vi "GUI_HTU_MultiCamBeamPointing1.vi"() -> ()   [LabVIEW 2020]
uses:
  Shared/GUI_Template/GUI_master/tcp_new_data_event.ctl
  Shared/GUI_Template/GUI_master/tcp new data cluster.ctl
  General GUIs/Device GUIs/GUI_Cameras/Controls/Crosshair type def.ctl
  <userlib>/_OpenG.lib/array/array.llb/Filter 1D Array with Scalar (String)__ogtk.vi
panel:
  out "x-y 8":dbl
  out "x-y 7":dbl
  out "x-y 6":dbl
  out "x-y 5":dbl
  out "x-y 4":dbl
  out "x-y 3":dbl
  out "x-y 2":dbl
  out "x-y":dbl
  out "String 8":string="x1\ny1\nx2\ny2"
  out "String 7":string="x1\ny1\nx2\ny2"
  out "String 6":string="x1\ny1\nx2\ny2"
  out "String 5":string="x1\ny1\nx2\ny2"
  out "String 4":string="x1\ny1\nx2\ny2"
  out "String 3":string="x1\ny1\nx2\ny2"
  out "String 2":string="x1\ny1\nx2\ny2"
  out "String":string="x1\ny1\nx2\ny2"
  in  "visibility":bool=TRUE
  out "appended array":string[](array[string]) caption="XH"
  out "appended array 6":string[](array[string]) caption="XH"
  out "appended array 8":string[](array[string]) caption="XH"
  out "appended array 4":string[](array[string]) caption="XH"
  in  "UDP error message":string
  out "tcp data event 2":T1
  out "error IO 2":errorcluster
  in  "Color Box":u32(colorbox)
  in  "TargetSize.Y::5":dbl=45.0 caption="y" min=2.0 max=3000.0 format="%#_6f"
  in  "TargetSize.X::5":dbl=47.0 caption="x" min=2.0 max=3000.0 format="%#_6f"
  in  "TargetSize.Y::4":dbl=45.0 caption="y" min=2.0 max=3000.0 format="%#_6f"
  in  "TargetSize.X::4":dbl=47.0 caption="x" min=2.0 max=3000.0 format="%#_6f"
  in  "TargetSize.Y::3":dbl=163.0 caption="y" min=2.0 max=3000.0 format="%#_6f"
  in  "TargetSize.X::3":dbl=152.0 caption="x" min=2.0 max=3000.0 format="%#_6f"
  in  "TargetSize.Y::2":dbl=74.0 caption="y" min=2.0 max=3000.0 format="%#_6f"
  in  "TargetSize.X::2":dbl=75.0 caption="x" min=2.0 max=3000.0 format="%#_6f"
  in  "active cams":string
  out "CCDs":string[](array[string])
  out "Cameras":T2
  in  "Target.Y::5":dbl=45.0 caption="y" min=0.0 max=2000.0 format="%#_6f"
  in  "Target.X::5":dbl=47.0 caption="x" min=0.0 max=2000.0 format="%#_6f"
  in  "Target.Y::4":dbl=45.0 caption="y" min=0.0 max=2000.0 format="%#_6f"
  in  "Target.X::4":dbl=47.0 caption="x" min=0.0 max=2000.0 format="%#_6f"
  in  "Target.Y::3":dbl=163.0 caption="y" min=0.0 max=2000.0 format="%#_6f"
  in  "Target.X::3":dbl=152.0 caption="x" min=0.0 max=2000.0 format="%#_6f"
  in  "Target.Y::2":dbl=74.0 caption="y" min=0.0 max=2000.0 format="%#_6f"
  in  "Target.X::2":dbl=75.0 caption="x" min=0.0 max=2000.0 format="%#_6f"
  out "error out":errorcluster
  in  "triggerdelay::5":dbl=0.001 caption="triggerdelay" min=10.0 max=1000000.0 format="%_4p"
  in  "triggerdelay::4":dbl=0.001 caption="triggerdelay" min=10.0 max=500000.0 format="%_4p"
  in  "triggerdelay::3":dbl=0.001 caption="triggerdelay" min=10.0 max=100000.0 format="%_4p"
  in  "triggerdelay::2":dbl=0.001 caption="triggerdelay" min=0.01 max=999000.0 format="%_4p"
  in  "trigger::5":bool caption="Trigger"
  in  "centroidy::5":dbl=0.001 caption="centroid y" min=0.0 max=0.0 format="%_4f"
  in  "centroidx::5":dbl=0.001 caption="centroid x" min=0.0 max=0.0 format="%_4f"
  in  "exposure::5":dbl=0.001 caption="exposure" min=1e-05 max=1.0 format="%_4p"
  out "image::5":T3(plugin-control) caption="HTT-MagCam-01"
  in  "GUIdevice 5":string="UC_BCaveIn"
  in  "trigger::4":bool caption="Trigger"
  in  "centroidy::4":dbl=0.001 caption="centroid y" min=0.0 max=0.0 format="%_4f"
  in  "centroidx::4":dbl=0.001 caption="centroid x" min=0.0 max=0.0 format="%_4f"
  in  "exposure::4":dbl=0.001 caption="exposure" min=5e-05 max=1.0 format="%_4p"
  out "image::4":T3(plugin-control) caption="HTT-MagCam-02"
  in  "GUIdevice 4":string="UC_DMSurface"
  in  "trigger::3":bool caption="Trigger"
  in  "centroidy::3":dbl=0.001 caption="centroid y" min=0.0 max=0.0 format="%_4f"
  in  "centroidx::3":dbl=0.001 caption="centroid x" min=0.0 max=0.0 format="%_4f"
  in  "exposure::3":dbl=0.001 caption="exposure" min=1e-05 max=1.0 format="%_4p"
  out "image::3":T3(plugin-control) caption="HTT-MagCam-03"
  in  "GUIdevice 3":string="UC_GratingMode"
  in  "trigger::2":bool caption="Trigger"
  in  "centroidy::2":dbl=0.001 min=0.0 max=0.0 format="%_4f"
  in  "centroidx::2":dbl=0.001 min=0.0 max=0.0 format="%_4f"
  in  "exposure::2":dbl=0.001 caption="exposure" min=5e-05 max=1.0 format="%_4p"
  out "image::2":T3(plugin-control) caption="HTT-MagCam-04"
  in  "GUIdevice 2":string="UC_TubeIn"
  out "tcp data event":T1
  in  "Refresh Button":bool caption="Update Crosshairs"
  in  "Select device":string(combo)="FrogHPD"
  in  "stop":bool
  in  "GUIdevice 1":string="HPD_CCD"
  # "XHair location"
  # "XHair location"
  # "XHair size"
  # "XHair size"
  # "XHair location"
  # "XHair size"
  # "XHair size"
  # "XHair location"
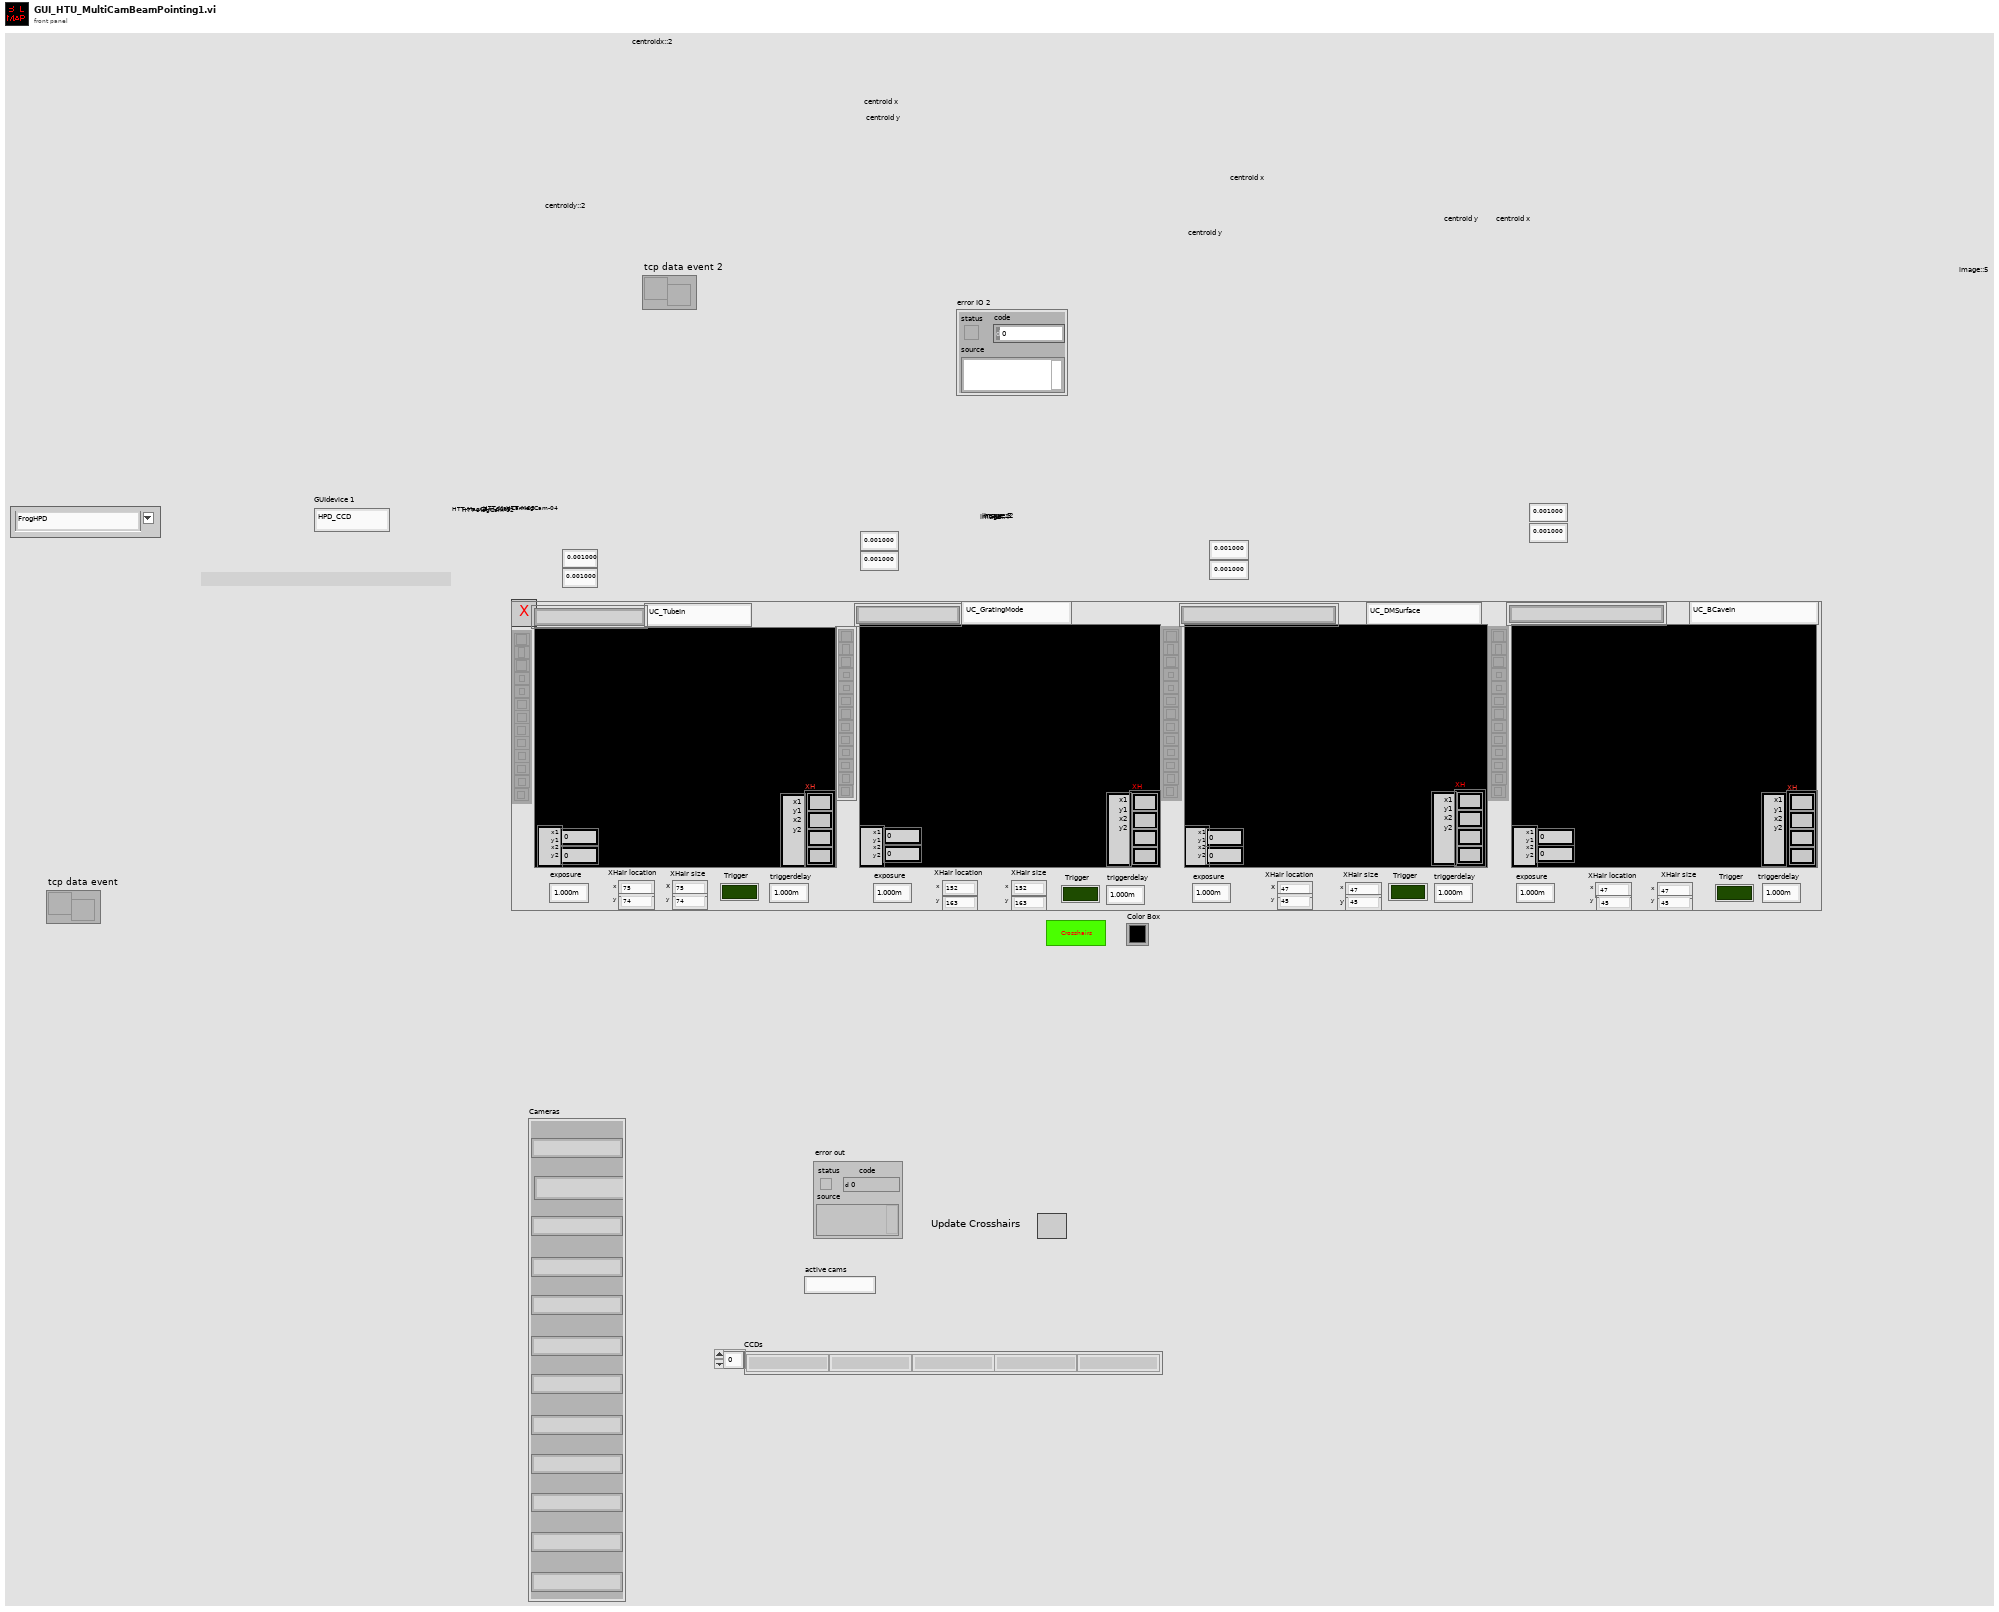
[diagram p1: front panel]
types:
  T1 = typedef "tcp_new_data_event.ctl" = refnum<user-event>
  T2 = cluster{"[0]":string, "[1]":string, "[2]":string, "[3]":string, "[4]":string, "[5]":string, "[6]":string, "[7]":string, "[8]":string, "[8] 2":string, "[8] 3":string, "[8] 4":string}
  T3 = typedef "IMAQ Image.ctl" = refnum<image>
  T4 = typedef "Image Type" = u32
  T5 = cluster{"Target.X::2":refnum<vi>, "Target.Y::2":refnum<vi>}
  T6 = cluster{"Target.X::3":refnum<vi>, "Target.Y::3":refnum<vi>}
  T7 = cluster{"Target.X::4":refnum<vi>, "Target.Y::4":refnum<vi>}
  T8 = cluster{"Target.X::5":refnum<vi>, "Target.Y::5":refnum<vi>}
  T9 = cluster{"TargetSize.X::2":refnum<vi>, "TargetSize.Y::2":refnum<vi>}
  T10 = cluster{"TargetSize.X::3":refnum<vi>, "TargetSize.Y::3":refnum<vi>}
  T11 = cluster{"TargetSize.X::4":refnum<vi>, "TargetSize.Y::4":refnum<vi>}
  T12 = cluster{"TargetSize.X::5":refnum<vi>, "TargetSize.Y::5":refnum<vi>}
  T13 = cluster{"Target.X::5":refnum<vi>, "Target.Y::5":refnum<vi>}[]
  T14 = cluster{"TargetSize.X::5":refnum<vi>, "TargetSize.Y::5":refnum<vi>}[]
  T15 = cluster{"[0]":string, "[1]":string, "[2]":string, "[3]":string, "[4]":string, "[5]":string, "[6]":string, "[7]":string, "[8]":string, "[9]":string, "[10]":string, "[11]":string}
  T16 = typedef "Crosshair type def.ctl" = cluster{"Draw":bool, "Target":cluster{"x":dbl, "y":dbl}, "Size":cluster{"x":dbl, "y":dbl}, "Angle":dbl, "Color":u32, "Thickness":u8, "CrosshairLabel":string}
  T17 = cluster{"Left":i32, "Top":i32, "Right":i32, "Bottom":i32}
  T18 = enum32{"invalid app kind", "Development System", "Run Time System", "Student Edition", "Embedded LabVIEW", "Evaluation", "Custom"}
  T19 = typedef "tcp new data cluster.ctl" = cluster{"EventEnum":enum16{"new data", "connection status update"}, "Device name":string}
  T20 = enum32{"Invalid", "Standard", "Closed", "Hidden", "Minimized", "Maximized"}
  T21 = cluster{"Core":cluster{"Current VI Reference":refnum<vi>, "Close Panel on Exit?":bool}, "Your Boolean data":bool, "active cams":string, "SuperGUI":cluster{"STOP queue":refnum<queue>, "SuperGUI ref":refnum<vi>}}
  T22 = cluster{"STOP queue":refnum<queue>, "SuperGUI ref":refnum<vi>}
  T23 = cluster{"Current VI Reference":refnum<vi>, "Close Panel on Exit?":bool}
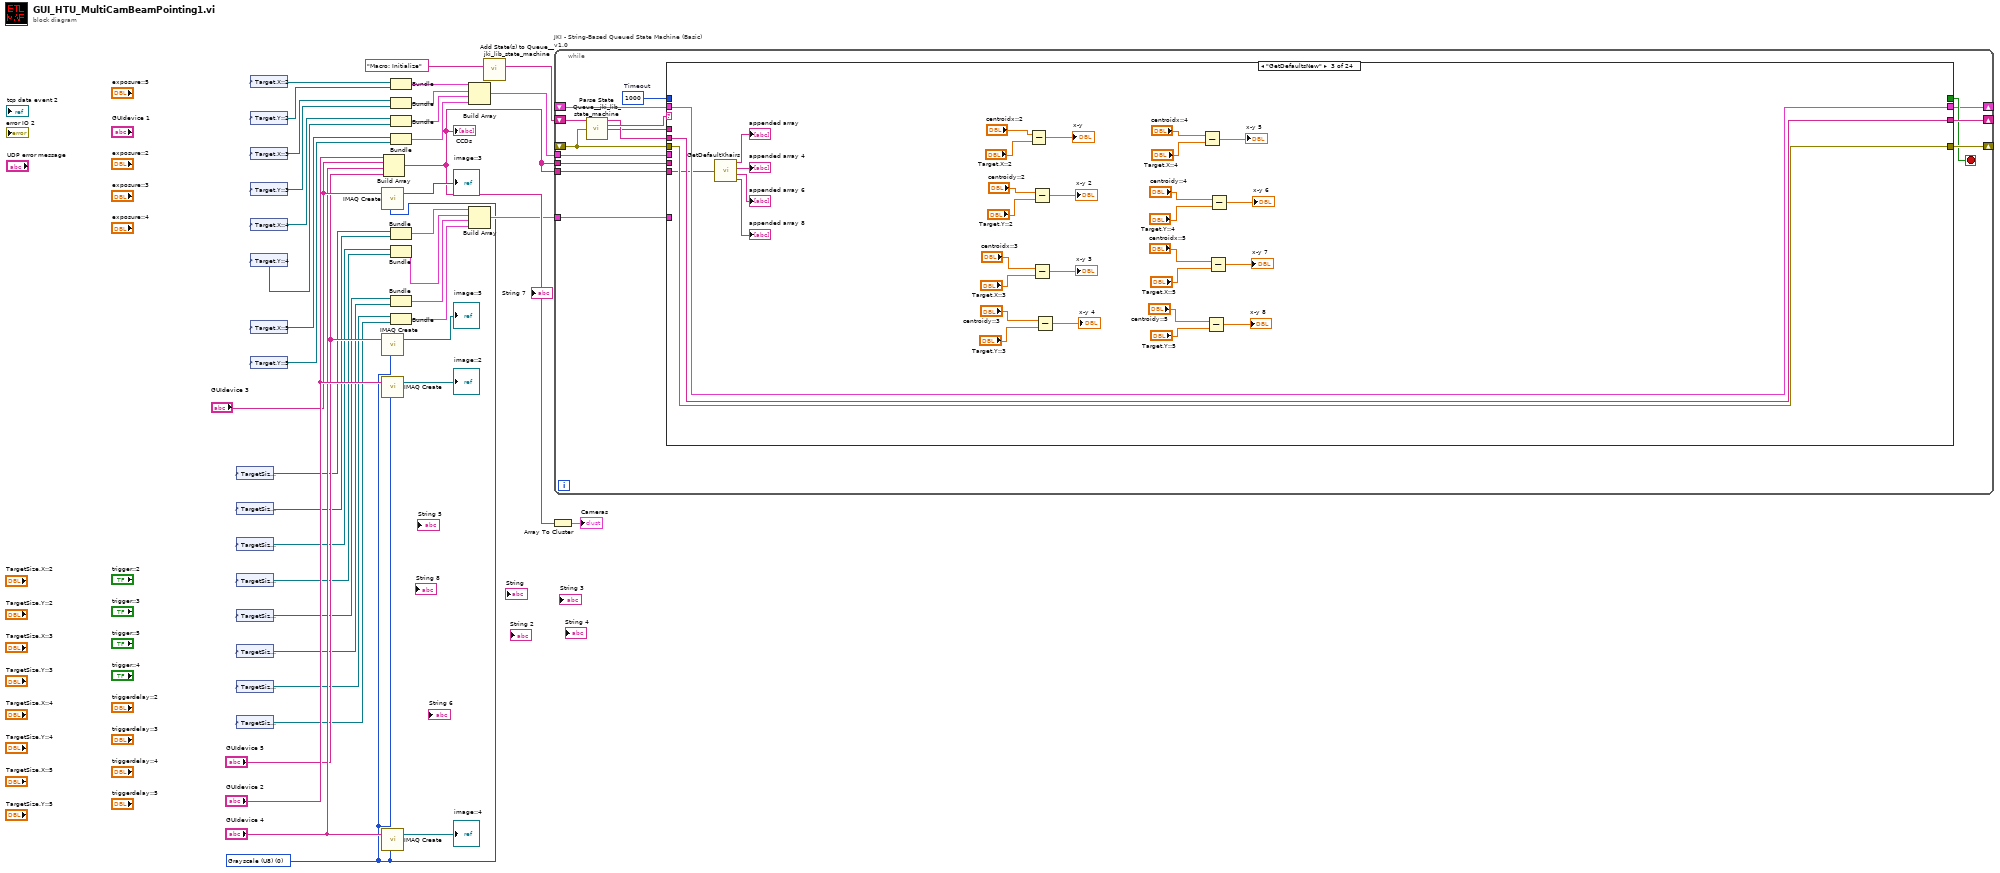
[diagram p0: block diagram]
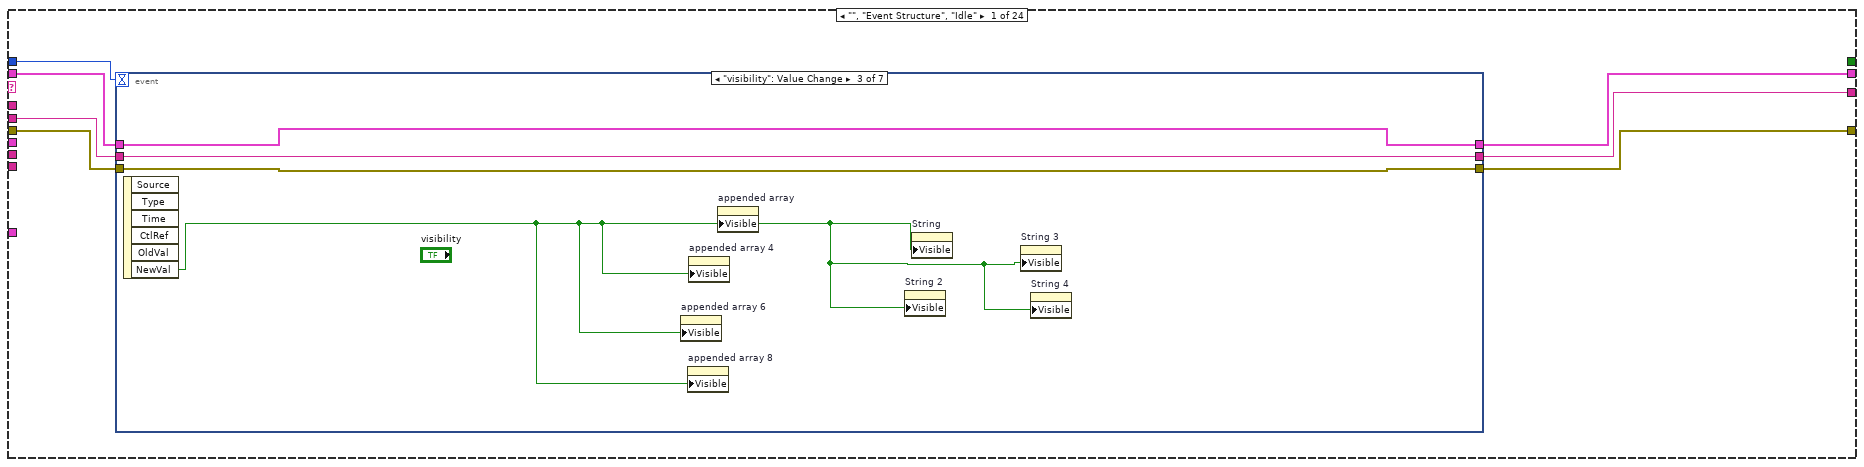
[diagram p2: hidden frame]
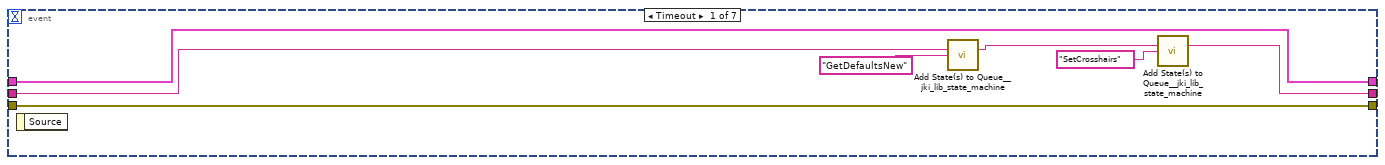
[diagram p3: hidden frame]
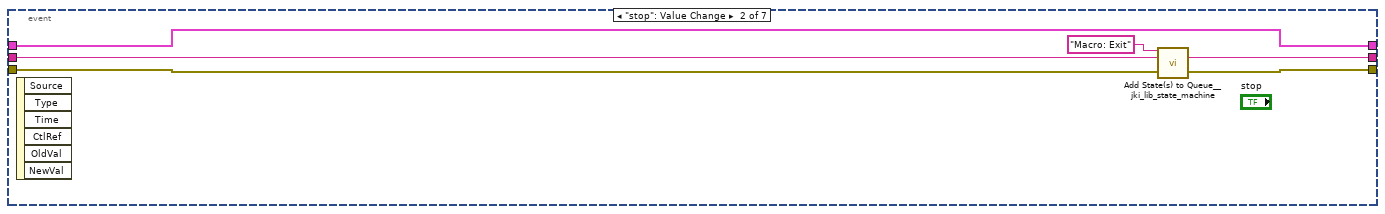
[diagram p4: hidden frame]
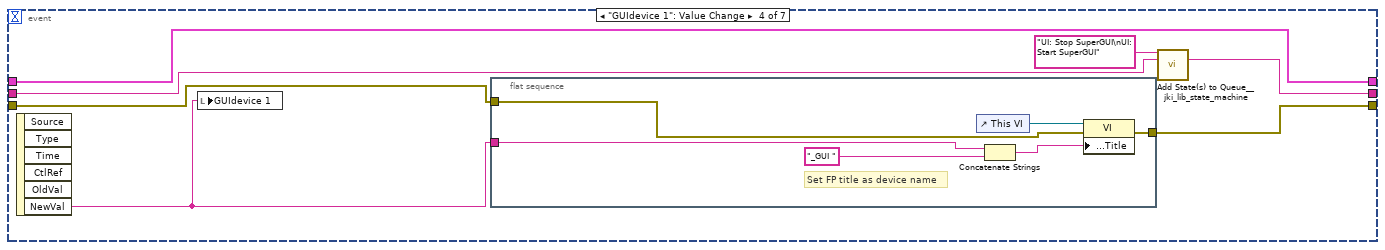
[diagram p5: hidden frame]
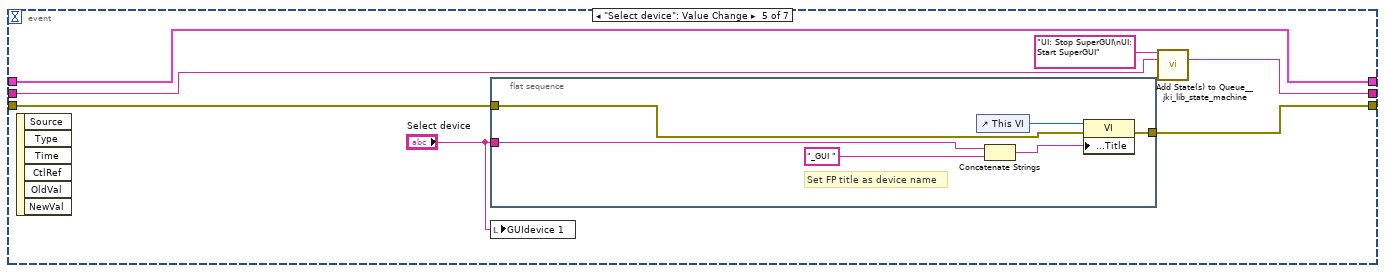
[diagram p6: hidden frame]
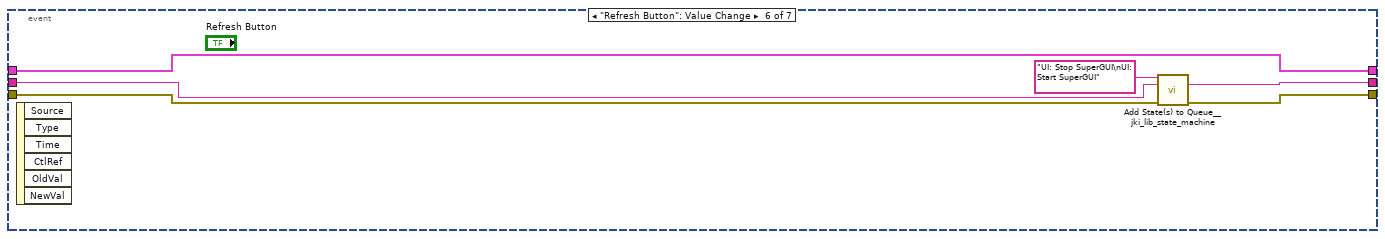
[diagram p7: hidden frame]
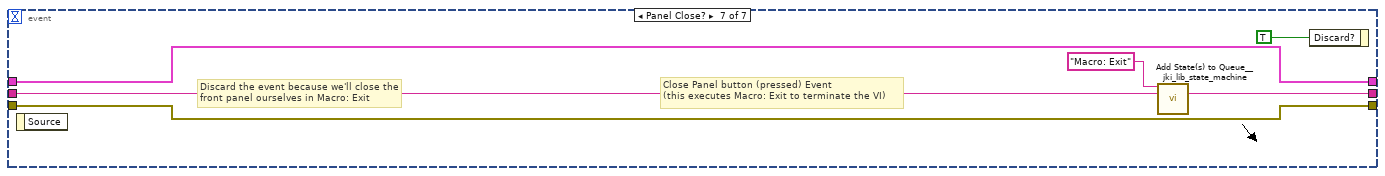
[diagram p8: hidden frame]
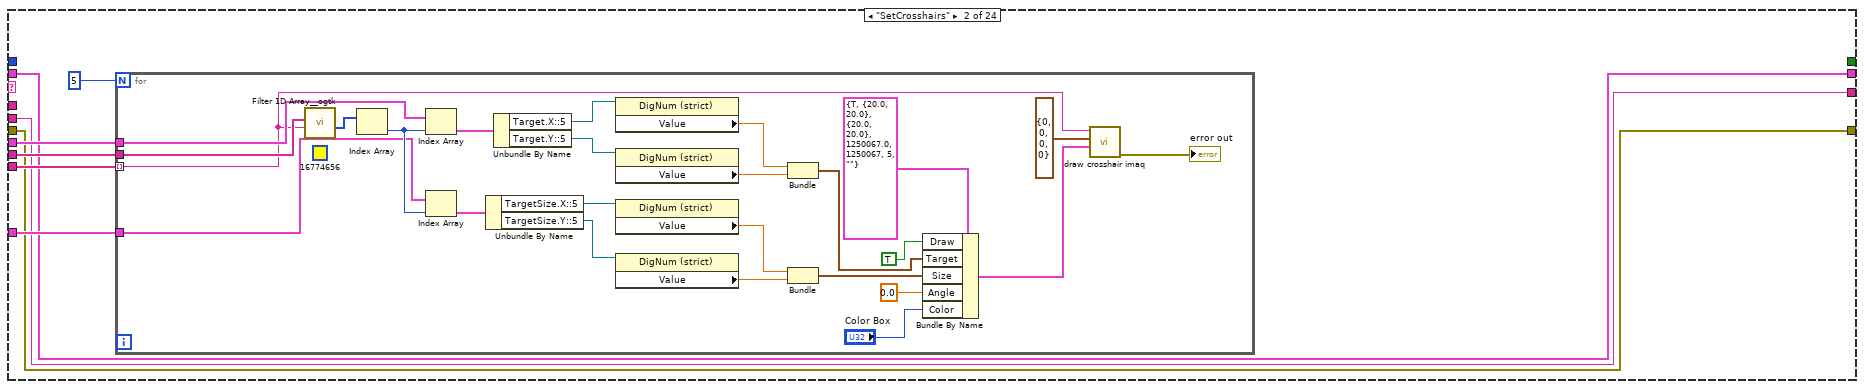
[diagram p9: hidden frame]
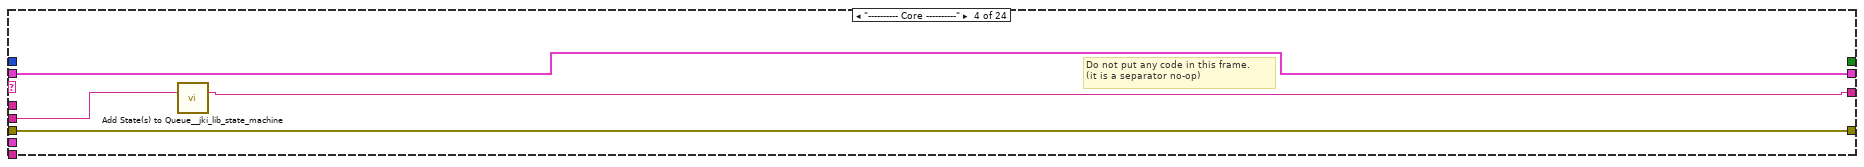
[diagram p10: hidden frame]
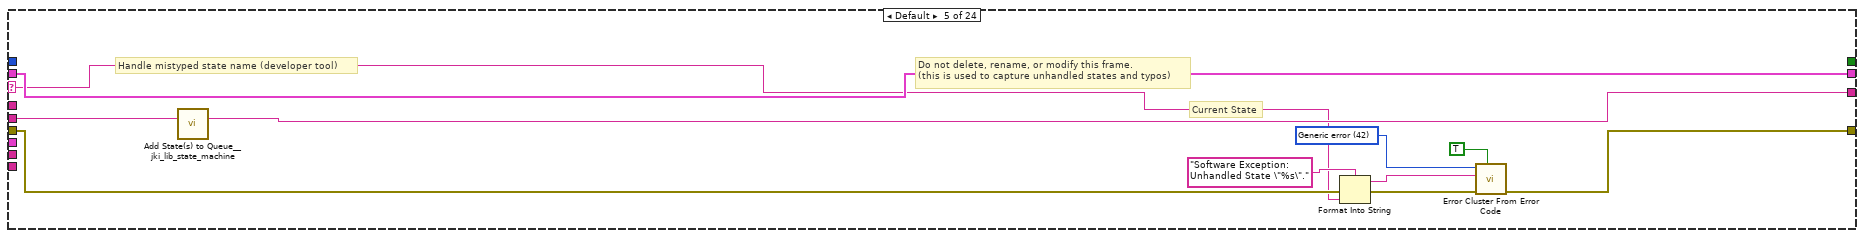
[diagram p11: hidden frame]
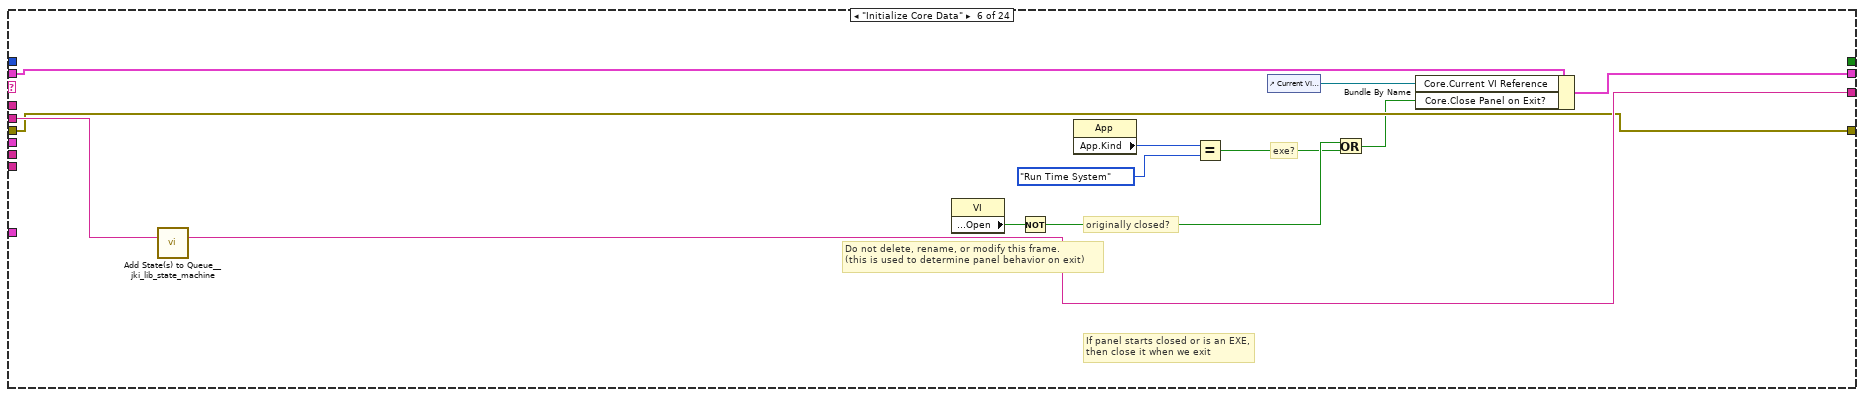
[diagram p12: hidden frame]
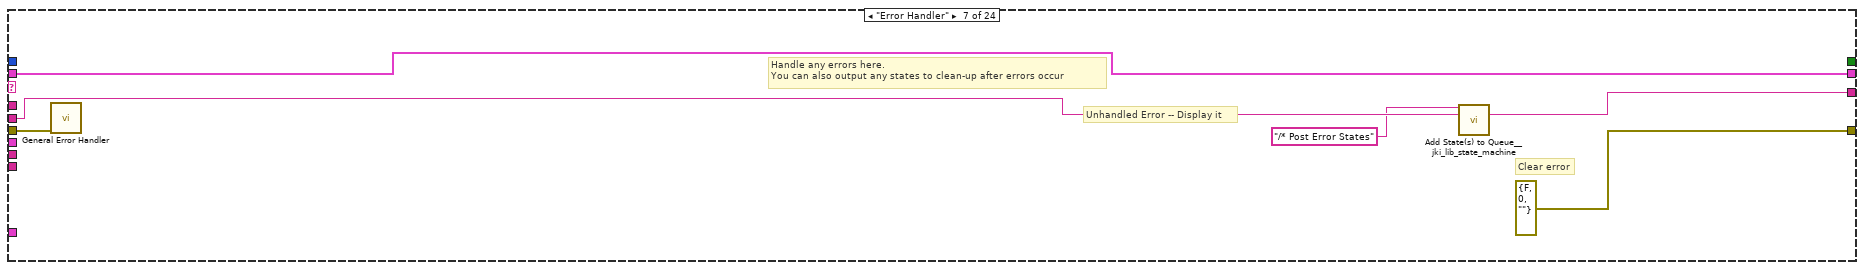
[diagram p13: hidden frame]
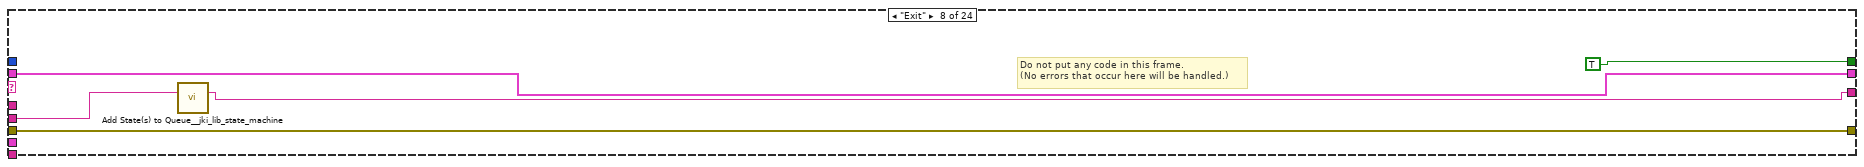
[diagram p14: hidden frame]
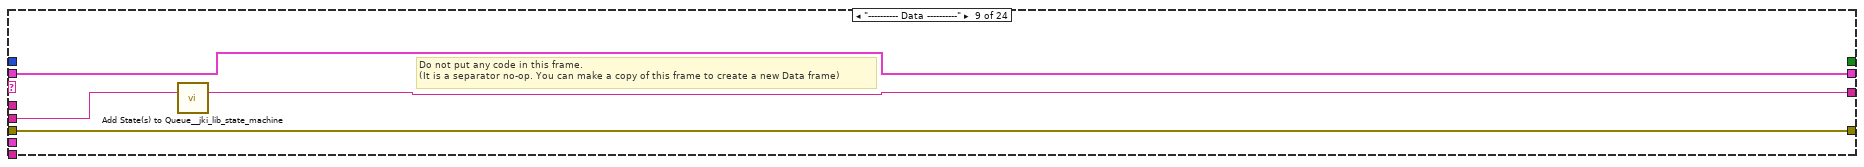
[diagram p15: hidden frame]
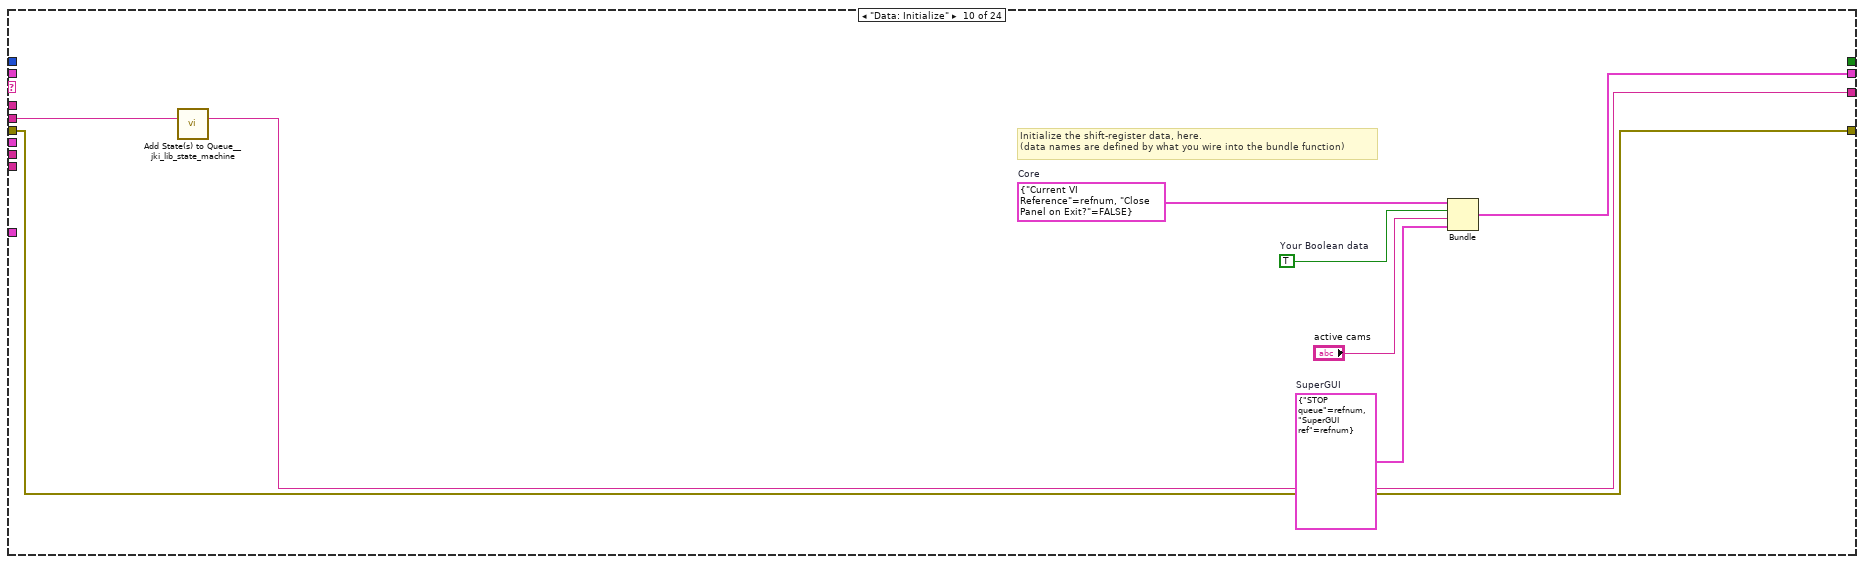
[diagram p16: hidden frame]
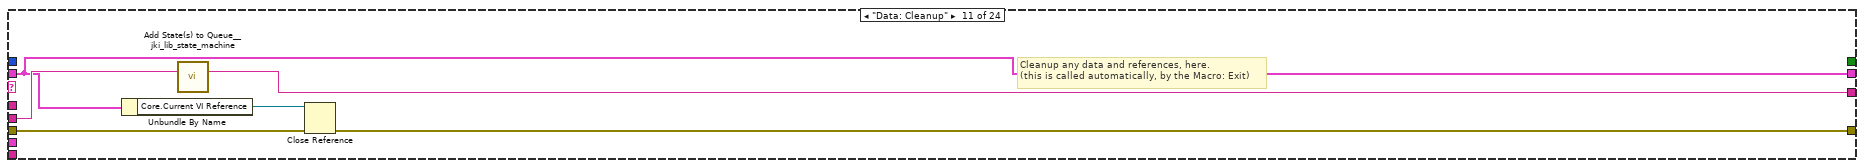
[diagram p17: hidden frame]
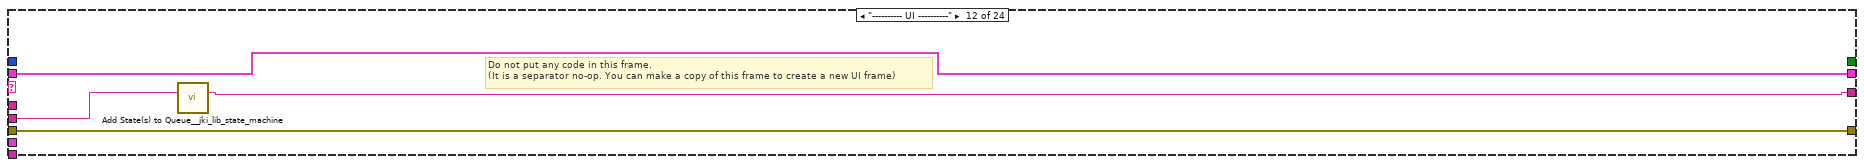
[diagram p18: hidden frame]
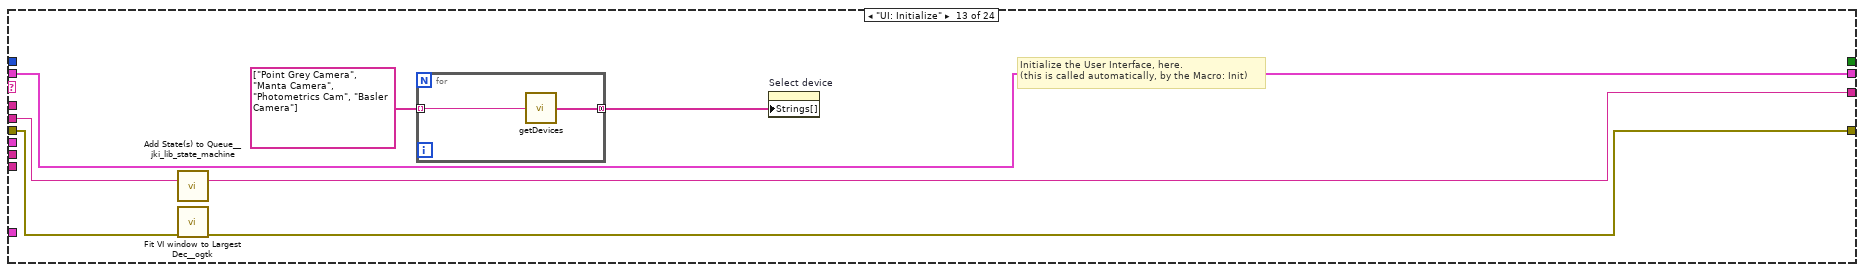
[diagram p19: hidden frame]
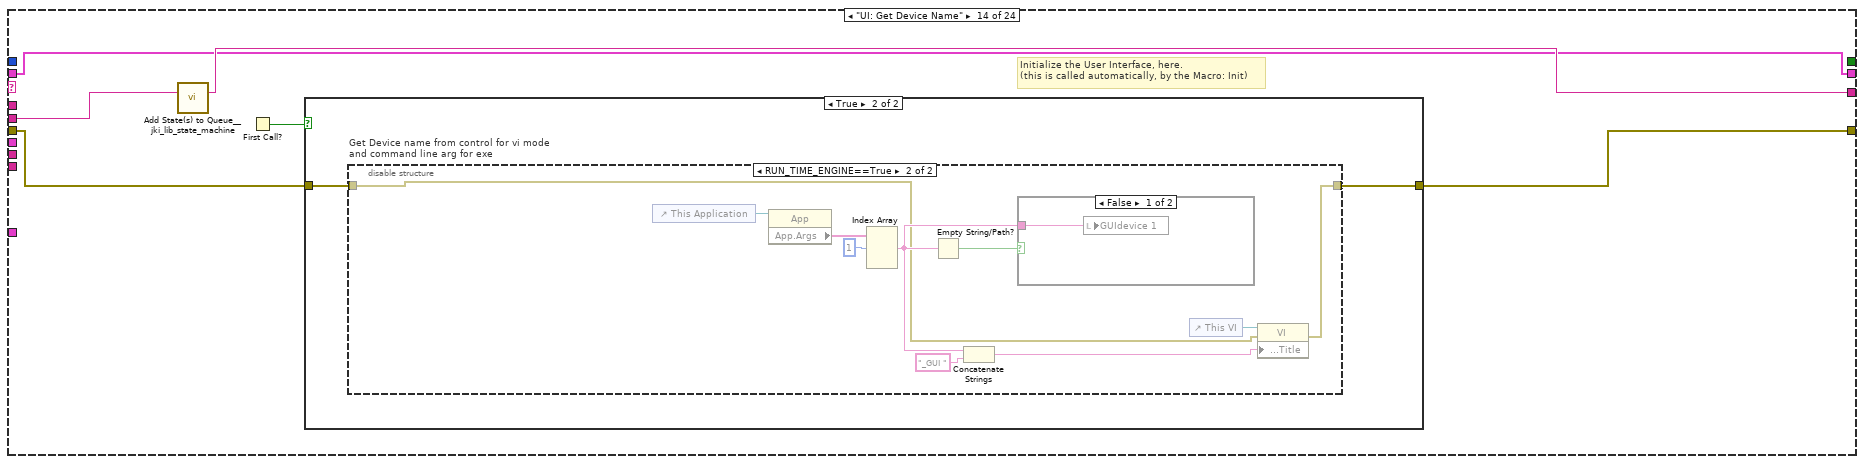
[diagram p20: hidden frame]
diagram:
  w1 = T4 0 items=["Grayscale (U8)", "Grayscale (I16)", "Grayscale (SGL)", "Complex (CSG)", "RGB (U32)", "HSL (U32)", "RGB (U64)", "Grayscale (U16)"] ("Image Type")
  n1 = control-ref of="TargetSize.X::2"() -> (w14:refnum<vi>)
  n2 = control-ref of="TargetSize.Y::2"() -> (w13:refnum<vi>)
  n3 = control-ref of="TargetSize.X::3"() -> (w12:refnum<vi>)
  n4 = control-ref of="TargetSize.Y::3"() -> (w11:refnum<vi>)
  n5 = control-ref of="TargetSize.X::4"() -> (w10:refnum<vi>)
  n6 = control-ref of="TargetSize.Y::4"() -> (w9:refnum<vi>)
  n7 = control-ref of="TargetSize.X::5"() -> (w8:refnum<vi>)
  n8 = control-ref of="TargetSize.Y::5"() -> (w7:refnum<vi>)
  n9 = control-ref of="Target.X::2"() -> (w33:refnum<vi>)
  n10 = control-ref of="Target.Y::2"() -> (w32:refnum<vi>)
  n11 = control-ref of="Target.X::3"() -> (w31:refnum<vi>)
  n12 = control-ref of="Target.Y::3"() -> (w30:refnum<vi>)
  n13 = control-ref of="Target.X::4"() -> (w29:refnum<vi>)
  n14 = control-ref of="Target.Y::4"() -> (w28:refnum<vi>)
  n15 = control-ref of="Target.X::5"() -> (w27:refnum<vi>)
  n16 = control-ref of="Target.Y::5"() -> (w26:refnum<vi>)
  n17 = call "IMAQ Create"("Image Name"="GUIdevice 3", "Image Type"=w1) -> ("New Image"=→"image::3":T3)  [unwired: 3 in, 1 out]
  n18 = call "IMAQ Create"("Image Name"="GUIdevice 5", "Image Type"=w1) -> ("New Image"=→"image::5":T3)  [unwired: 3 in, 1 out]
  n19 = call "IMAQ Create"("Image Name"="GUIdevice 2", "Image Type"=w1) -> ("New Image"=→"image::2":T3)  [unwired: 3 in, 1 out]
  n20 = call "IMAQ Create"("Image Name"="GUIdevice 4", "Image Type"=w1) -> ("New Image"=→"image::4":T3)  [unwired: 3 in, 1 out]
  n21 = Build Array("GUIdevice 2", "GUIdevice 3", "GUIdevice 4", "GUIdevice 5") -> (w15:string[])
  "CCDs" <- w15
  n22 = Bundle("Target.X::2"=w33, "Target.Y::2"=w32) -> (w25:T5)  [unwired: 1 in]
  n23 = Bundle("Target.X::3"=w31, "Target.Y::3"=w30) -> (w24:T6)  [unwired: 1 in]
  n24 = Bundle("Target.X::4"=w29, "Target.Y::4"=w28) -> (w22:T7)  [unwired: 1 in]
  n25 = Bundle("Target.X::5"=w27, "Target.Y::5"=w26) -> (w23:T8)  [unwired: 1 in]
  n26 = Bundle("TargetSize.X::2"=w14, "TargetSize.Y::2"=w13) -> (w6:T9)  [unwired: 1 in]
  n27 = Bundle("TargetSize.X::3"=w12, "TargetSize.Y::3"=w11) -> (w5:T10)  [unwired: 1 in]
  n28 = Bundle("TargetSize.X::4"=w10, "TargetSize.Y::4"=w9) -> (w3:T11)  [unwired: 1 in]
  n29 = Bundle("TargetSize.X::5"=w8, "TargetSize.Y::5"=w7) -> (w4:T12)  [unwired: 1 in]
  n30 = Build Array(w25, w24, w22, w23) -> (w21:T13)
  n31 = Build Array(w6, w5, w3, w4) -> (w2:T14)
  n32 = call <vilib>:"Add State(s) to Queue__jki_lib_state_machine.vi"("State(s) in (\"\")"="Macro: Initialize") -> ("States Out"=w39:string)  [unwired: 14 in]
  n33 = Array To Cluster(array=w15) -> (cluster=→"Cameras":T15)
  n34 = while "JKI - String-Based Queued State Machine (Basic) v1.0" {
    shift-right: [w47] -> _
    shift-left: _ -> [w44]
    shift-right: [w50] -> _
    shift-left: _ -> [w45]
    shift-right: [w49] -> _
    shift-left: w39 -> [w51]
    tunnel: w21 -> [w41]
    tunnel: w15 -> [w42]
    tunnel: w15 -> [w43]
    tunnel: w2 -> [w40]
    stop <- w48 stop-if-true
    w46 = 1000  # Timeout
    n35 = call <vilib>:"Parse State Queue__jki_lib_state_machine.vi"("State Queue"=w51, "Error In (no error)"=w45) -> ("Remaining States"=w53:string, "Current State"=w54:string, "Arguments"=w52:string)  [unwired: 11 in]
    n36 = case shown="\"GetDefaultsNew\"" w54 {
      selector: w54 -> [_ _ _ _ w184 _ _ _ _ _ _ _ _ _ _ _ _ _ _ _ _ _ _ _]
      tunnel: w53 -> [w61 w117 w178 w183 w188 w206 w212 w217 w221 w229 w235 w239 w246 w254 w289 w297 w303 w314 w340 w345 w355 w359 w363 w367]
      tunnel: w52 -> [_ _ _ _ _ _ _ _ _ _ _ _ _ _ _ _ w298 w308 _ _ _ _ _ _]
      tunnel: w44 -> [w59 w118 w179 w180 w186 w197 w209 w215 w218 _ w230 w236 w244 w252 w280 w292 w301 w310 w337 w342 w352 w356 w360 w364]
      tunnel: [w58 w116 w177 w181 w190 w203 errorcluster {"status"=FALSE, "code"=0, "source"=""} ("error out") w214 w219 w226 w231 w237 w242 w249 w273 w290 w299 w311 w338 w343 w353 w357 w361 w365] -> w50
      tunnel: w45 -> [w57 w116 w177 w181 w189 w203 w208 w214 w219 w226 w232 w237 w243 w250 w274 w291 w300 w312 w338 w343 w353 w357 w361 w365]
      tunnel: [w60 w117 w178 w182 w187 w205 w211 w216 w220 w228 w234 w238 w245 w253 w288 w296 w302 w313 w339 w344 w354 w358 w362 w366] -> w49
      tunnel: [_ _ _ _ _ _ _ TRUE _ _ _ _ _ _ _ _ _ _ _ _ _ _ _ _] -> w48
      tunnel: [w56 w118 w179 w180 w186 w204 w209 w215 w218 w227 w230 w236 w244 w252 w279 w292 w301 w310 w337 w342 w352 w356 w360 w364] -> w47
      tunnel: w46 -> [w55 _ _ _ _ _ _ _ _ _ _ _ _ _ _ _ _ _ _ _ _ _ _ _]
      tunnel: w43 -> [_ w120 w176 _ _ _ _ _ _ _ _ _ _ _ _ _ _ _ _ _ _ _ _ _]
      tunnel: w42 -> [_ w121 _ _ _ _ _ _ _ _ _ _ _ _ _ _ _ _ _ _ _ _ _ _]
      tunnel: w41 -> [_ w122 _ _ _ _ _ _ _ _ _ _ _ _ _ _ _ _ _ _ _ _ _ _]
      tunnel: w40 -> [_ w119 _ _ _ _ _ _ _ _ _ _ _ _ _ _ _ _ _ _ _ _ _ _]
      frame "", "Event Structure", "Idle" {
        n37 = event shown="[2] \"visibility\": Value Change" {
          selector: _ -> [_ _ _ _ _ _ _]
          dyn-events: _ -> [_ _ _ _ _ _ _]
          timeout: w55 -> [_ _ _ _ _ _ _]
          tunnel: w61 -> [w64 w71 w75 w81 w93 w106 w114]
          tunnel: [w68 w70 w75 w80 w92 w105 w113] -> w60
          tunnel: w59 -> [w66 w73 w77 w84 w97 w108 w111]
          tunnel: [w67 w72 w76 w82 w95 w107 w112] -> w58
          tunnel: w57 -> [w67 w72 w76 w83 w96 w107 w112]
          tunnel: [w66 w73 w77 w84 w97 w108 w111] -> w56
          event Timeout {
            n38 = event-data() -> ()  [unwired: 1 in, 1 out]
            n39 = call <vilib>:"Add State(s) to Queue__jki_lib_state_machine.vi"("State(s) in (\"\")"=w64, "State(s) at Back (\"\")"="GetDefaultsNew") -> ("States Out"=w62:string)  [unwired: 13 in]
            n40 = call <vilib>:"Add State(s) to Queue__jki_lib_state_machine.vi"("State(s) in (\"\")"=w62, "State(s) at Back (\"\")"="SetCrosshairs") -> ("States Out"=w68:string)  [unwired: 13 in]
          }
          event "stop": Value Change {
            n41 = event-data() -> ()  [unwired: 1 in, 6 out]
            n42 = call <vilib>:"Add State(s) to Queue__jki_lib_state_machine.vi"("State(s) in Front (\"\")"="Macro: Exit", "State(s) in (\"\")"=w71) -> ("States Out"=w70:string)  [unwired: 13 in]
          }
          event "visibility": Value Change {
            n43 = event-data() -> ("NewVal"=w74:bool)  [unwired: 1 in, 5 out]
            n44 = property on="appended array 6" class="Arr (strict)"("Visible"=w74) -> ()  [unwired: 2 in, 2 out]
            n45 = property on="appended array 8" class="Arr (strict)"("Visible"=w74) -> ()  [unwired: 2 in, 2 out]
            n46 = property on="appended array 4" class="Arr (strict)"("Visible"=w74) -> ()  [unwired: 2 in, 2 out]
            n47 = property on="appended array" class="Arr (strict)"("Visible"=w74) -> ()  [unwired: 2 in, 2 out]
            n48 = property on="String 2" class="Str"("Visible"=w74) -> ()  [unwired: 2 in, 2 out]
            n49 = property on="String" class="Str"("Visible"=w74) -> ()  [unwired: 2 in, 2 out]
            n50 = property on="String 3" class="Str"("Visible"=w74) -> ()  [unwired: 2 in, 2 out]
            n51 = property on="String 4" class="Str"("Visible"=w74) -> ()  [unwired: 2 in, 2 out]
          }
          event "GUIdevice 1": Value Change {
            n52 = event-data() -> ("NewVal"=w78:string)  [unwired: 1 in, 5 out]
            n53 = local write "GUIdevice 1"(w78) -> ()
            n54 = flat-sequence {
              tunnel: [w87] -> w82
              tunnel: w83 -> [w86]
              tunnel: w78 -> [w85]
              frame #0 {
                # "Set FP title as device name"
                n55 = control-ref of="This VI"() -> (w90:refnum<vi>)
                n56 = Concatenate Strings(w85, "_GUI ") -> (w89:string)
                n57 = property class="VI"(reference=w90, error in=w86, "Front Panel.Title"=w89) -> (error out=w87:errorcluster)  [unwired: 1 out]
              }
            }
            n58 = call <vilib>:"Add State(s) to Queue__jki_lib_state_machine.vi"("State(s) in Front (\"\")"="UI: Stop SuperGUI\nUI: Start SuperGUI", "State(s) in (\"\")"=w81) -> ("States Out"=w80:string)  [unwired: 13 in]
          }
          event "Select device": Value Change {
            n59 = event-data() -> ()  [unwired: 1 in, 6 out]
            n60 = flat-sequence {
              tunnel: [w100] -> w95
              tunnel: w96 -> [w99]
              tunnel: "Select device" -> [w98]
              frame #0 {
                # "Set FP title as device name"
                n61 = control-ref of="This VI"() -> (w103:refnum<vi>)
                n62 = Concatenate Strings(w98, "_GUI ") -> (w102:string)
                n63 = property class="VI"(reference=w103, error in=w99, "Front Panel.Title"=w102) -> (error out=w100:errorcluster)  [unwired: 1 out]
              }
            }
            n64 = local write "GUIdevice 1"("Select device") -> ()
            n65 = call <vilib>:"Add State(s) to Queue__jki_lib_state_machine.vi"("State(s) in Front (\"\")"="UI: Stop SuperGUI\nUI: Start SuperGUI", "State(s) in (\"\")"=w93) -> ("States Out"=w92:string)  [unwired: 13 in]
          }
          event "Refresh Button": Value Change {
            n66 = event-data() -> ()  [unwired: 1 in, 6 out]
            n67 = call <vilib>:"Add State(s) to Queue__jki_lib_state_machine.vi"("State(s) in Front (\"\")"="UI: Stop SuperGUI\nUI: Start SuperGUI", "State(s) in (\"\")"=w106) -> ("States Out"=w105:string)  [unwired: 13 in]
          }
          event Panel Close? {
            # "Discard the event because we'll close the front panel ourselves in Macro: Exit"
            # "Close Panel button (pressed) Event\n(this executes Macro: Exit to terminate the VI)"
            n68 = event-data() -> ()  [unwired: 1 in, 1 out]
            n69 = call <vilib>:"Add State(s) to Queue__jki_lib_state_machine.vi"("State(s) in Front (\"\")"="Macro: Exit", "State(s) in (\"\")"=w114) -> ("States Out"=w113:string)  [unwired: 13 in]
            n70 = event-data("Discard?"=TRUE) -> ()  [unwired: 1 in, 1 out]
          }
        }
      }
      frame "SetCrosshairs" {
        n71 = for {
          N: 5 -> [_]
          tunnel: w121 -> [w126]
          tunnel: w122 -> [w125]
          tunnel: w119 -> [w124]
          tunnel: w120 -> [w123] mode=indexing
          (unwired) u32 16774656 ("Color")
          n72 = call-poly <userlib>:"Filter 1D Array__ogtk.vi"("items to filter"=w123, "array"=w126) -> ("filtered item indices"=w130:i32[])  [unwired: 4 in, 1 out]
          n73 = Index Array(array=w130) -> (element=w133:i32)  [unwired: 1 in]
          n74 = Index Array(array=w125, index=w133) -> (element=w131:T8)
          n75 = Index Array(array=w124, index=w133) -> (element=w134:T12)
          n76 = Unbundle By Name(w134) -> ("TargetSize.X::5"=w135:refnum<vi>, "TargetSize.Y::5"=w136:refnum<vi>)
          n77 = Unbundle By Name(w131) -> ("Target.X::5"=w128:refnum<vi>, "Target.Y::5"=w129:refnum<vi>)
          n78 = property class="DigNum (strict)"(reference=w128) -> ("Value"=w142:dbl)  [unwired: 1 in, 2 out]
          n79 = property class="DigNum (strict)"(reference=w129) -> ("Value"=w143:dbl)  [unwired: 1 in, 2 out]
          n80 = property class="DigNum (strict)"(reference=w135) -> ("Value"=w137:dbl)  [unwired: 1 in, 2 out]
          n81 = property class="DigNum (strict)"(reference=w136) -> ("Value"=w138:dbl)  [unwired: 1 in, 2 out]
          n82 = Bundle("Value"=w142, "Value"=w143) -> (w144:cluster{"Value":dbl, "Value":dbl})  [unwired: 1 in]
          n83 = Bundle("Value"=w137, "Value"=w138) -> (w145:cluster{"Value":dbl, "Value":dbl})  [unwired: 1 in]
          n84 = Bundle By Name(cluster=T16 {"Draw"=TRUE, "Target"={"x"=20.0, "y"=20.0}, "Size"={"x"=20.0, "y"=20.0}, "Angle"=1250067.0, "Color"=1250067, "Thickness"=5, "CrosshairLabel"=""} ("Crosshair"), "Draw"=TRUE, "Target"=w144, "Size"=w145, "Angle"=0.0, "Color"="Color Box") -> (w140:T16)
          n85 = call "draw crosshair imaq.vi"("Crosshair"=w140, "Bounding Rectangle"=T17 {"Left"=0, "Top"=0, "Right"=0, "Bottom"=0}, "image in"=w123) -> ("error out"=→"error out":errorcluster)  [unwired: 7 in, 1 out]
        }
      }
      frame "GetDefaultsNew" {
        n86 = call "GetDefaultXhairs.vi"("appended array 2"=w176) -> ("appended array"=→"appended array":string[], "appended array 4"=→"appended array 4":string[], "appended array 6"=→"appended array 6":string[], "appended array 8"=→"appended array 8":string[])
        n87 = Subtract(x="centroidx::2", y="Target.X::2") -> (x-y=→"x-y":dbl)
        n88 = Subtract(x="centroidy::2", y="Target.Y::2") -> (x-y=→"x-y 2":dbl)
        n89 = Subtract(x="centroidx::3", y="Target.X::3") -> (x-y=→"x-y 3":dbl)
        n90 = Subtract(x="centroidy::3", y="Target.Y::3") -> (x-y=→"x-y 4":dbl)
        n91 = Subtract(x="centroidx::4", y="Target.X::4") -> (x-y=→"x-y 5":dbl)
        n92 = Subtract(x="centroidy::5", y="Target.Y::5") -> (x-y=→"x-y 8":dbl)
        n93 = Subtract(x="centroidx::5", y="Target.X::5") -> (x-y=→"x-y 7":dbl)
        n94 = Subtract(x="centroidy::4", y="Target.Y::4") -> (x-y=→"x-y 6":dbl)
      }
      frame "---------- Core ----------" {
        # "Do not put any code in this frame.\n(it is a separator no-op)"
        n95 = call <vilib>:"Add State(s) to Queue__jki_lib_state_machine.vi"("State(s) in (\"\")"=w183) -> ("States Out"=w182:string)  [unwired: 14 in]
      }
      frame Default {
        w193 = 42 items=["No error", "Argument error", "Memory is full", "Out of zone", "End of file", "File already open", "Generic file I/O error", "File not found", "File permission error", "Disk is full", "Duplicate path", "Too many files open", "System feature not enabled", "Resource file not found", "Cannot add resource", "Resource not found", "Image not found", "Image memory error", "Pen does not exist", "Config type invalid", "Config token not found", "Config parse error", "Config memory error", "Bad external code format", "Bad external code offset", "External code not present", "Null window", "Destroy window error", "Null menu", "Print aborted", "Bad print record", "Print driver error", "Windows error during printing", "Memory error during printing", "Print dialog error", "Generic print error", "Invalid device refnum", "Device not found", "Device parameter error", "Device unit error", "Cannot open device", "Device call aborted", "Generic error", "Cancelled by user", "Object ID too low", "Object ID too high", "Object not in heap", "Unknown heap", "Unknown object (invalid DefProc)", "Unknown object (DefProc not in table)", "Message out of range", "Invalid (null) method", "Unknown message", "Manager call not supported", "Bad address", "Network operation in progress", "Network operation timed out", "Connection is busy", "Network attribute not supported", "Network error", "Address in use", "System out of memory", "Connection aborted", "Connection refused", "Not connected", "Already connected", "Connection closed", "Initialization error (interapplication manager)", "Bad occurrence", "Wait on unbound occurrence handler", "Occurrence queue overflow", "Datalog type conflict", "Unused", "Unrecognized type (interapplication manager)", "Memory corrupt", "Failed to make temporary DLL", "Old CIN version", "Drag socket not found", "Failed to load drop-object", "Failed to register OLE object", "Failed to release OLE object", "Format specifier type mismatch", "Unknown format specifier", "Too few format specifiers", "Too many format specifiers", "Scan failed", "Newer CIN version", "Error converting to variant", "Runtime menu error", "Password tampered", "Variant attribute not found", "Incompatible variant data type", "Event data is not available", "Event Store is not present", "Occurrence is not found", "Event Queue is not created", "Event info is not available", "Refnum passed is NULL", "Error retrieving Class GUID", "Error retrieving CoClass GUID", "Error retrieving TypeLib GUID.", "Bad built application magic bytes.", "Specific driver is different from the specific driver associated with the Logical Name.", "There is no session opened to the class driver.", "Max Error", "MAX - Error with config objects", "MAX - Error loading configuration", "MAX - Group not supported"]
        # "Current State"
        # "Do not delete, rename, or modify this frame.\n(this is used to capture unhandled states and typos)"
        # "Handle mistyped state name (developer tool)"
        n96 = call <vilib>:"Add State(s) to Queue__jki_lib_state_machine.vi"("State(s) in (\"\")"=w188) -> ("States Out"=w187:string)  [unwired: 14 in]
        n97 = Format Into String(format string="Software Exception: Unhandled State \"%s\"." ("message"), error in=w189, w184) -> (resulting string=w192:string, error out=w191:errorcluster)  [unwired: 1 in]
        n98 = call <vilib>:"Error Cluster From Error Code.vi"("show call chain? (False)"=TRUE, "error in (no error)"=w191, "error message (\"\")"=w192, "error code (0)"=w193) -> ("error out"=w190:errorcluster)  [unwired: 5 in]
      }
      frame "Initialize Core Data" {
        # "Do not delete, rename, or modify this frame.\n(this is used to determine panel behavior on exit)"
        # "originally closed?"
        # "exe?"
        # "If panel starts closed or is an EXE, then close it when we exit"
        n99 = call <vilib>:"Add State(s) to Queue__jki_lib_state_machine.vi"("State(s) in (\"\")"=w206) -> ("States Out"=w205:string)  [unwired: 14 in]
        n100 = property class="VI"() -> ("Front Panel.Open"=w202:bool)  [unwired: 2 in, 2 out]
        n101 = Not(x=w202) -> (.not. x?=w199:bool)
        n102 = property class="App"() -> ("App.Kind"=w201:T18)  [unwired: 2 in, 2 out]
        n103 = Equal?(x=w201, y=T18."Run Time System" ("Application:Kind")) -> (x = y?=w198:bool)
        n104 = control-ref of="Current VI Reference"() -> (w195:refnum<vi>)
        n105 = Or(x=w199, y=w198) -> (x .or. y?=w196:bool)
        n106 = Bundle By Name(cluster=w197, "Core.Current VI Reference"=w195, "Core.Close Panel on Exit?"=w196) -> (w204:T21)
      }
      frame "Error Handler" {
        # "Unhandled Error -- Display it"
        # "Handle any errors here.\nYou can also output any states to clean-up after errors occur"
        # "Clear error"
        n107 = call <vilib>:"General Error Handler.vi"("error in (no error)"=w208) -> ()  [unwired: 10 in, 5 out]
        n108 = call <vilib>:"Add State(s) to Queue__jki_lib_state_machine.vi"("State(s) in Front (\"\")"="/* Post Error States", "State(s) in (\"\")"=w212) -> ("States Out"=w211:string)  [unwired: 13 in]
      }
      frame "Exit" {
        # "Do not put any code in this frame.\n(No errors that occur here will be handled.)"
        n109 = call <vilib>:"Add State(s) to Queue__jki_lib_state_machine.vi"("State(s) in (\"\")"=w217) -> ("States Out"=w216:string)  [unwired: 14 in]
      }
      frame "---------- Data ----------" {
        # "Do not put any code in this frame.\n(It is a separator no-op. You can make a copy of this frame to create a new Data frame)"
        n110 = call <vilib>:"Add State(s) to Queue__jki_lib_state_machine.vi"("State(s) in (\"\")"=w221) -> ("States Out"=w220:string)  [unwired: 14 in]
      }
      frame "Data: Initialize" {
        w222 = T22 {"STOP queue"=refnum, "SuperGUI ref"=refnum}  # SuperGUI
        w223 = T23 {"Current VI Reference"=refnum, "Close Panel on Exit?"=FALSE}  # Core
        w225 = TRUE  # Your Boolean data
        # "Initialize the shift-register data, here.\n(data names are defined by what you wire into the bundle function)"
        n111 = call <vilib>:"Add State(s) to Queue__jki_lib_state_machine.vi"("State(s) in (\"\")"=w229) -> ("States Out"=w228:string)  [unwired: 14 in]
        n112 = Bundle("Core"=w223, "Your Boolean data"=w225, "active cams"="active cams", "SuperGUI"=w222) -> (w227:T21)  [unwired: 1 in]
      }
      frame "Data: Cleanup" {
        # "Cleanup any data and references, here.\n(this is called automatically, by the Macro: Exit)"
        n113 = Unbundle By Name(w230) -> ("Core.Current VI Reference"=w233:refnum<vi>)
        n114 = call <vilib>:"Add State(s) to Queue__jki_lib_state_machine.vi"("State(s) in (\"\")"=w235) -> ("States Out"=w234:string)  [unwired: 14 in]
        n115 = Close Reference(reference=w233, error in (no error)=w232) -> (error out=w231:errorcluster)
      }
      frame "---------- UI ----------" {
        # "Do not put any code in this frame.\n(It is a separator no-op. You can make a copy of this frame to create a new UI frame)"
        n116 = call <vilib>:"Add State(s) to Queue__jki_lib_state_machine.vi"("State(s) in (\"\")"=w239) -> ("States Out"=w238:string)  [unwired: 14 in]
      }
      frame "UI: Initialize" {
        # "Initialize the User Interface, here.\n(this is called automatically, by the Macro: Init)"
        n117 = call <vilib>:"Add State(s) to Queue__jki_lib_state_machine.vi"("State(s) in (\"\")"=w246) -> ("States Out"=w245:string)  [unwired: 14 in]
        n118 = call <userlib>:"Fit VI window to Largest Dec__ogtk.vi"("error in (no error)"=w243) -> ("error out"=w242:errorcluster)  [unwired: 5 in, 1 out]
        n119 = for {
          tunnel: string[] ["Point Grey Camera", "Manta Camera", "Photometrics Cam", "Basler Camera"] -> [w248] mode=indexing
          tunnel: [w247] -> w240 mode=concatenating
          n120 = call "getDevices.vi"("Device Class"=w248) -> ("All Devices"=w247:string[])
        }
        n121 = property on="Select device" class="CmbBox"("Strings[]"=w240) -> ()  [unwired: 2 in, 2 out]
      }
      frame "UI: Get Device Name" {
        # "Initialize the User Interface, here.\n(this is called automatically, by the Macro: Init)"
        n122 = call <vilib>:"Add State(s) to Queue__jki_lib_state_machine.vi"("State(s) in (\"\")"=w254) -> ("States Out"=w253:string)  [unwired: 14 in]
        n123 = First Call?() -> (First Call?: T/F=w251:bool)
        n124 = case shown="True" w251 {
          tunnel: w250 -> [w255 w257]
          tunnel: [w255 w256] -> w249
          frame False {
          }
          frame True {
            n125 = disable-structure "Get Device name from control for vi mode\nand command line arg for exe" shown="RUN_TIME_ENGINE==True" {
              disable-tunnel: w257 -> [w258 w260]
              disable-tunnel: [w258 w259] -> w256
              frame condition #0 (active) {
              }
              frame condition #1 {
                n126 = control-ref of="This Application"() -> (w268:refnum<vi>)
                n127 = property class="App"(reference=w268) -> ("App.Args"=w267:string[])  [unwired: 1 in, 2 out]
                n128 = Index Array(array=w267, index #1=1 ("index")) -> (element #1=w261:string)  [unwired: 2 in, 2 out]
                n129 = Empty String/Path?(string/path=w261) -> (empty?=w265:bool)
                n130 = Concatenate Strings(w261, "_GUI ") -> (w263:string)
                n131 = case shown="False" w265 {
                  tunnel: w261 -> [w269 _]
                  frame False {
                    n132 = local write "GUIdevice 1"(w269) -> ()
                  }
                  frame True {
                  }
                }
                n133 = control-ref of="This VI"() -> (w264:refnum<vi>)
                n134 = property class="VI"(reference=w264, error in=w260, "Front Panel.Title"=w263) -> (error out=w259:errorcluster)  [unwired: 1 out]
              }
            }
          }
        }
      }
      frame "UI: Start SuperGUI" {
        # "create stop queue for supergui and its clones"
        # "x100 abort will be dependent on caller VI\nx80 abort will be independent of caller vi, this will abort vi when labview is closed."
        # "Start SuperGUI asynchronous way"
        n135 = vi-ref "GUI_Master_subvi_reentrant_queues.vi"() -> (w272:refnum<vi>)
        n136 = property class="VI"(reference=w272) -> ("Path"=w271:path)  [unwired: 1 in, 2 out]
        n137 = control-ref of="This Application"() -> (w278:refnum<vi>)
        n138 = Open VI Reference(type specifier VI Refnum (for type only)=refnum<vi> refnum, vi path=w271, options=256) -> (vi reference=w287:refnum<vi>, error out=w286:errorcluster)  [unwired: 3 in]
        n139 = Create User Event(user event datatype=T19 {"EventEnum"=enum."new data", "Device name"="Device name"} ("New Event"), error in=w274) -> (user event=w275:refnum<user-event>, error out=w281:errorcluster)
        "tcp data event" <- w275
        n140 = control-ref of="This VI"() -> (w277:refnum<vi>)
        n141 = register-events(w275) -> ()  [unwired: 2 in, 2 out]
        n142 = call "supergui create stop queue.vi"() -> ("STOP Queue out"=w283:refnum<queue>)  [unwired: 11 in]
        n143 = Current VI's Menubar() -> (w276:refnum<k9>)
        n144 = call-by-ref "Start Asynchronous Call"(reference=w287, error in=w286, "STOP Queue in"=w283, "This Application"=w278, 8:"error in (no error)"=w281, "tcp data event"=w275, "Caller menu reference"=w276, "Caller VI ref"=w277) -> (reference out=w270:refnum<vi>, error out=w273:errorcluster)  [unwired: 5 in, 1 out]
        n145 = Bundle By Name(cluster=w280, "SuperGUI.SuperGUI ref"=w270, "SuperGUI.STOP queue"=w283) -> (w279:T21)
        n146 = call <vilib>:"Add State(s) to Queue__jki_lib_state_machine.vi"("State(s) in (\"\")"=w289) -> ("States Out"=w288:string)  [unwired: 14 in]
      }
      frame "UI: Stop SuperGUI" {
        # "Stop Supergui Clone and wait until it exit properly"
        n147 = call <vilib>:"Add State(s) to Queue__jki_lib_state_machine.vi"("State(s) in (\"\")"=w297) -> ("States Out"=w296:string)  [unwired: 14 in]
        n148 = Unbundle By Name(w292) -> ("SuperGUI.SuperGUI ref"=w294:refnum<vi>, "SuperGUI.STOP queue"=w293:refnum<queue>)
        n149 = Release Queue(queue=w293, error in (no error)=w291) -> (error out=w295:errorcluster)  [unwired: 1 in, 2 out]
        n150 = call-by-ref "Wait On Asynchronous Call"(reference=w294, error in=w295) -> ("error out"=w290:errorcluster)  [unwired: 11 in, 2 out]
      }
      frame "UI: Cursor Set" {
        # "Argument"
        # "Set and Unset Cursor Busy.\n(Usage: \"UI: Cursor Set >> Busy|Idle\")"
        n151 = call <vilib>:"Add State(s) to Queue__jki_lib_state_machine.vi"("State(s) in (\"\")"=w303) -> ("States Out"=w302:string)  [unwired: 14 in]
        n152 = case shown="\"Idle\", Default" w298 {
          tunnel: w300 -> [w305 w307]
          tunnel: [w304 w306] -> w299
          frame "Idle", Default {
            n153 = call <vilib>:"Unset Busy.vi"("error in (no error)"=w305) -> ("error out"=w304:errorcluster)  [unwired: 10 in]
          }
          frame "Busy" {
            n154 = call <vilib>:"Set Busy.vi"("error in (no error)"=w307) -> ("error out"=w306:errorcluster)  [unwired: 9 in, 1 out]
          }
        }
      }
      frame "UI: Front Panel State" {
        # "Argument"
        # "Set Front Panel Open or Closed\n(Usage: \"UI: Front Panel State >> Open|Close\")"
        n155 = call <vilib>:"Add State(s) to Queue__jki_lib_state_machine.vi"("State(s) in (\"\")"=w314) -> ("States Out"=w313:string)  [unwired: 14 in]
        n156 = Unbundle By Name(w310) -> ("Core.Current VI Reference"=w309:refnum<vi>)
        n157 = case shown="\"Open\", Default" w308 {
          tunnel: w312 -> [w318 w331]
          tunnel: [w320 w332] -> w311
          tunnel: w309 -> [w319 w329]
          frame "Open", Default {
            n158 = property class="VI"(reference=w319, error in=w318) -> (reference out=w316:refnum<vi>, error out=w317:errorcluster, "Front Panel.Open"=w315:bool)
            n159 = case shown="False" w315 {
              tunnel: [w323 w326] -> w320
              tunnel: w317 -> [w322 w326]
              tunnel: w316 -> [w321 _]
              frame False {
                n160 = invoke class="VI" method="FP.Open"(reference=w321, error in=w322, "Activate"=TRUE, "State"=T20."Standard") -> (error out=w323:errorcluster)  [unwired: 1 in, 4 out]
              }
              frame True {
              }
            }
          }
          frame "Close" {
            n161 = property class="VI"(reference=w329, error in=w331) -> (reference out=w328:refnum<vi>, error out=w330:errorcluster, "Front Panel.Open"=w327:bool)
            n162 = case shown="True" w327 {
              tunnel: [w333 w336] -> w332
              tunnel: w330 -> [w333 w335]
              tunnel: w328 -> [_ w334]
              frame False {
              }
              frame True {
                n163 = invoke class="VI" method="FP.Close"(reference=w334, error in=w335) -> (error out=w336:errorcluster)  [unwired: 1 in, 2 out]
              }
            }
          }
        }
      }
      frame "---------- Macro ----------" {
        # "Do not put any code in this frame.\n(It is a separator no-op. You can make a copy of this frame to create a new Macro frame)"
        n164 = call <vilib>:"Add State(s) to Queue__jki_lib_state_machine.vi"("State(s) in (\"\")"=w340) -> ("States Out"=w339:string)  [unwired: 14 in]
      }
      frame "Macro: Initialize" {
        # "Initialization Macro\n(This is called once, when the VI starts)"
        n165 = call <vilib>:"Add State(s) to Queue__jki_lib_state_machine.vi"("State(s) in Front (\"\")"="Data: Initialize\nInitialize Core Data\nUI: Initialize\nUI: Get Device Name\nUI: Start SuperGUI\nUI: Front Panel State >> Open", "State(s) in (\"\")"=w345) -> ("States Out"=w344:string)  [unwired: 13 in]
      }
      frame "Macro: Exit" {
        # "Exit Macro\n(This is called once, when the VI exits)"
        n166 = Unbundle By Name(w352) -> ("Core.Close Panel on Exit?"=w351:bool)
        n167 = Select(t="UI: Front Panel State >> Close", s=w351, f="") -> (s? t:f=w348:string)
        n168 = call <vilib>:"Add State(s) to Queue__jki_lib_state_machine.vi"("State(s) in (\"\")"=w348, "State(s) at Back (\"\")"="Data: Cleanup\nExit") -> ("States Out"=w346:string)  [unwired: 13 in]
        n169 = call <vilib>:"Add State(s) to Queue__jki_lib_state_machine.vi"("State(s) in Front (\"\")"=w346, "State(s) in (\"\")"=w355) -> ("States Out"=w354:string)  [unwired: 13 in]
      }
      frame "---------- New Category ----------" {
        # "Template Separator\n(You can make a copy of, or modify, this frame)"
        n170 = call <vilib>:"Add State(s) to Queue__jki_lib_state_machine.vi"("State(s) in (\"\")"=w359) -> ("States Out"=w358:string)  [unwired: 14 in]
      }
      frame "New Category: 1" {
        # "Your code here.\n(You can make a copy of, or modify, this frame)"
        n171 = call <vilib>:"Add State(s) to Queue__jki_lib_state_machine.vi"("State(s) in (\"\")"=w363) -> ("States Out"=w362:string)  [unwired: 14 in]
      }
      frame "New Category: 2" {
        # "Your code here.\n(You can make a copy of, or modify, this frame)"
        n172 = call <vilib>:"Add State(s) to Queue__jki_lib_state_machine.vi"("State(s) in (\"\")"=w367) -> ("States Out"=w366:string)  [unwired: 14 in]
      }
    }
  }
